vi "Write Tool Rack.vi"(8 "error in (no error)":errorcluster, 10 "Tool Rack":T1, 11 "WorkTable Class in":refnum<class "WorkTable Class.lvclass">) -> (0 "error out":errorcluster, 3 "WorkTable Class out":refnum<class "WorkTable Class.lvclass">)   [LabVIEW 2011, in "WorkTable Class.lvclass"]
uses:
  WorkTable Class.lvclass
  Type Definitions/Worktable_Tool Rack.ctl
  WorkTable Class.lvclass/WorkTable Class.ctl
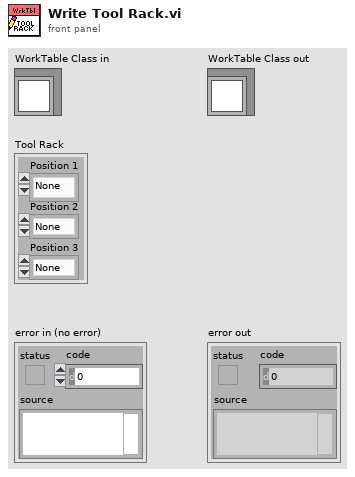
[diagram p1: front panel]
types:
  T1 = typedef "Worktable_Tool Rack.ctl" = cluster{"Position 1":enum16{"None", "Grabber", "Picker", "Tool Setter"}, "Position 2":enum16{"None", "Grabber", "Picker", "Tool Setter"}, "Position 3":enum16{"None", "Grabber", "Picker", "Tool Setter"}}
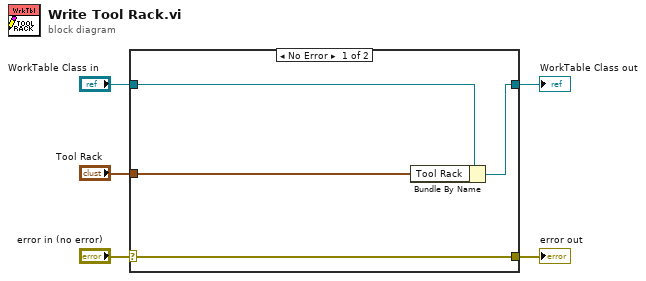
[diagram p0: block diagram]
diagram:
  n1 = case shown="No Error" "error in (no error)" {
    selector: "error in (no error)" -> [w9 w10]
    tunnel: [w9 w10] -> w4
    tunnel: [w7 w11] -> w2
    tunnel: "WorkTable Class in" -> [w8 w11]
    tunnel: "Tool Rack" -> [w6 _]
    frame No Error {
      n2 = Bundle By Name(cluster=w8, "Tool Rack"=w6) -> (w7:refnum<class "WorkTable Class.lvclass">)
    }
    frame Error {
    }
  }
  "error out" <- w4
  "WorkTable Class out" <- w2
